vi "Clean Up Actor.vi"(8 "error in (no error)":errorcluster, 11 "Car Wash Station Sequencer in":refnum<class "Car Wash Station Sequencer.lvclass">) -> (0 "error out":errorcluster, 3 "Car Wash Station Sequencer out":refnum<class "Car Wash Station Sequencer.lvclass">)   [LabVIEW 2016, in "CLD Exam - Car Wash.lvlib" / "Car Wash Station Sequencer.lvclass"]
doc: "--\nCopyright © 2017 Composed SystemsI All rights reserved.\n\nAuthor: Jon McBee <jon.mcbee@composed.io>\n\nThis library is provided \"AS IS\" ,WITHOUT WARRANTIES OR\nCONDITIONS OF ANY KIND, either express or implied.\n\nComposed Systems -- composed.io\n\nStream 0.0.1.1\nJon McBee - Composed Systems\nCopyright (c) 2017, Composed Systems"
uses:
  Car Wash Station Sequencer.lvclass
  D:/Repos/Stream/software/Mediator/Classes/Mediated Actor/Mediated Actor.lvclass
  Mediator/Classes/Message Broker Interface/Message Broker Interface.lvclass
  Mediator/Classes/Mediated Synchronous Actor/Mediated Synchronous Actor.lvclass
  Mediator/Classes/Mediated Actor/Mediated Actor.lvclass
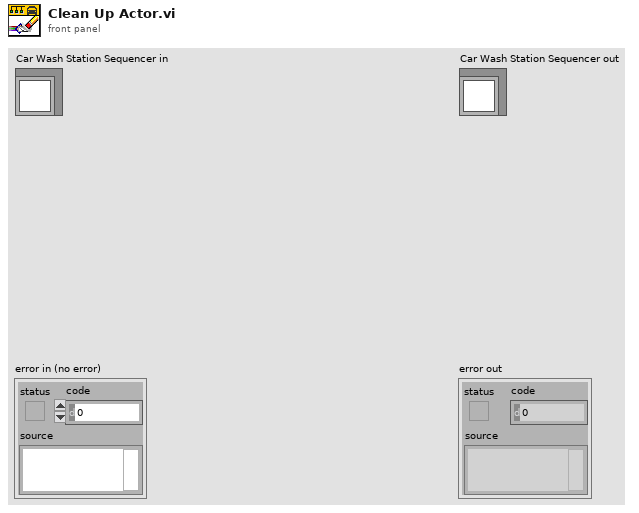
[diagram p1: front panel]
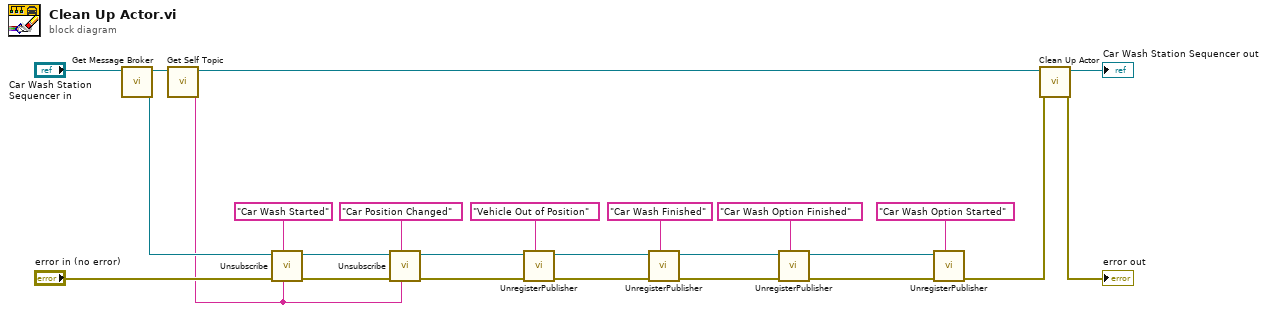
[diagram p0: block diagram]
diagram:
  n1 = call "Get Message Broker.vi"("Mediated Actor in"="Car Wash Station Sequencer in") -> ("Message Broker"=w14:refnum<class "Message Broker Interface.lvclass">, "Mediated Actor out"=w23:refnum<class "Car Wash Station Sequencer.lvclass">)  [unwired: 9 in]
  n2 = call "Get Self Topic.vi"("Mediated Actor in"=w23) -> ("Topic.Self"=w13:string, "Mediated Actor out"=w21:refnum<class "Car Wash Station Sequencer.lvclass">)  [unwired: 9 in]
  n3 = call-dynamic "Unsubscribe.vi"("Subscriber Name"=w13, "Topic Name"="Car Wash Started", "error in (no error)"="error in (no error)", "Message Broker Interface in"=w14) -> ("error out"=w17:errorcluster, "Message Broker Interface out"=w18:refnum<class "Message Broker Interface.lvclass">)  [unwired: 6 in]
  n4 = call-dynamic "Unsubscribe.vi"("Subscriber Name"=w13, "Topic Name"="Car Position Changed", "error in (no error)"=w17, "Message Broker Interface in"=w18) -> ("error out"=w11:errorcluster, "Message Broker Interface out"=w12:refnum<class "Message Broker Interface.lvclass">)  [unwired: 6 in]
  n5 = call-dynamic "UnregisterPublisher.vi"("Topic Name"="Vehicle Out of Position", "error in (no error)"=w11, "Message Broker Interface in"=w12) -> ("error out"=w8:errorcluster, "Message Broker Interface out"=w9:refnum<class "Message Broker Interface.lvclass">)  [unwired: 7 in]
  n6 = call-dynamic "UnregisterPublisher.vi"("Topic Name"="Car Wash Finished", "error in (no error)"=w8, "Message Broker Interface in"=w9) -> ("error out"=w5:errorcluster, "Message Broker Interface out"=w6:refnum<class "Message Broker Interface.lvclass">)  [unwired: 7 in]
  n7 = call-dynamic "UnregisterPublisher.vi"("Topic Name"="Car Wash Option Finished", "error in (no error)"=w5, "Message Broker Interface in"=w6) -> ("error out"=w2:errorcluster, "Message Broker Interface out"=w3:refnum<class "Message Broker Interface.lvclass">)  [unwired: 7 in]
  n8 = call-dynamic "UnregisterPublisher.vi"("Topic Name"="Car Wash Option Started", "error in (no error)"=w2, "Message Broker Interface in"=w3) -> ("error out"=w1:errorcluster)  [unwired: 7 in, 1 out]
  n9 = call-parent "Clean Up Actor.vi"("error in (no error)"=w1, "Mediated Actor in"=w21) -> ("error out"=→"error out":errorcluster, "Mediated Actor out"=→"Car Wash Station Sequencer out":refnum<class "Car Wash Station Sequencer.lvclass">)  [unwired: 8 in]
